vi "FG Error Counter.vi"(10 "count error":bool, 11 "reset to 0":bool) -> (2 "number of errors":i32)   [LabVIEW 2013]
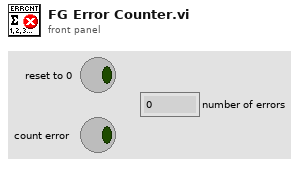
[diagram p1: front panel]
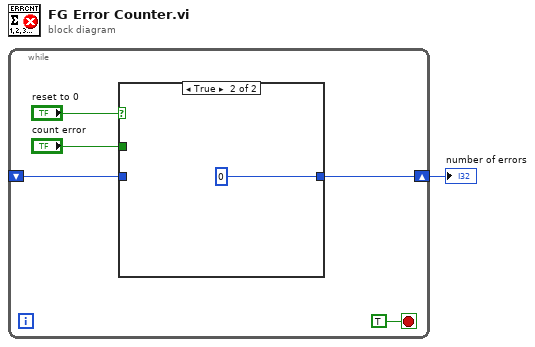
[diagram p0: block diagram]
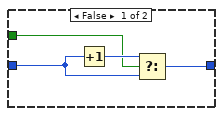
[diagram p2: hidden frame]
diagram:
  n1 = while {
    shift-right: [w4] -> w1
    shift-left: _ -> [w5]
    stop <- TRUE stop-if-true
    n2 = case shown="True" "reset to 0" {
      tunnel: w5 -> [w9 _]
      tunnel: [w8 0] -> w4
      tunnel: "count error" -> [w7 _]
      frame False {
        n3 = Increment(x=w9) -> (x+1=w10:i32)
        n4 = Select(t=w10, s=w7, f=w9) -> (s? t:f=w8:i32)
      }
      frame True {
      }
    }
  }
  "number of errors" <- w1
